vi "test TCX read (installed 71).vi"() -> ()   [LabVIEW 2011] (continued)
xmlns=\"http://www.garmin.com/xmlschemas/ActivityExtension/v2\"><Watts>102</Watts></TPX></Extensions></Trackpoint><Trackpoint><Time>2008-03-03T23:20:02Z</Time><Position><LatitudeDegrees>35.874903</LatitudeDegrees><LongitudeDegrees>-78.936135</LongitudeDegrees></Position><AltitudeMeters>84.253</AltitudeMeters><DistanceMeters>19044.637</DistanceMeters><Cadence>79</Cadence><Extensions><TPX xmlns=\"http://www.garmin.com/xmlschemas/ActivityExtension/v2\"><Watts>106</Watts></TPX></Extensions></Trackpoint><Trackpoint><Time>2008-03-03T23:20:03Z</Time><Position><LatitudeDegrees>35.874904</LatitudeDegrees><LongitudeDegrees>-78.936208</LongitudeDegrees></Position><AltitudeMeters>84.253</AltitudeMeters><DistanceMeters>19051.244</DistanceMeters><Cadence>79</Cadence><Extensions><TPX xmlns=\"http://www.garmin.com/xmlschemas/ActivityExtension/v2\"><Watts>107</Watts></TPX></Extensions></Trackpoint><Trackpoint><Time>2008-03-03T23:20:04Z</Time><Position><LatitudeDegrees>35.874906</LatitudeDegrees><LongitudeDegrees>-78.936282</LongitudeDegrees></Position><AltitudeMeters>84.253</AltitudeMeters><DistanceMeters>19057.943</DistanceMeters><Cadence>80</Cadence><Extensions><TPX xmlns=\"http://www.garmin.com/xmlschemas/ActivityExtension/v2\"><Watts>102</Watts></TPX></Extensions></Trackpoint><Trackpoint><Time>2008-03-03T23:20:05Z</Time><Position><LatitudeDegrees>35.874910</LatitudeDegrees><LongitudeDegrees>-78.936356</LongitudeDegrees></Position><AltitudeMeters>84.253</AltitudeMeters><DistanceMeters>19064.650</DistanceMeters><Cadence>80</Cadence><Extensions><TPX xmlns=\"http://www.garmin.com/xmlschemas/ActivityExtension/v2\"><Watts>102</Watts></TPX></Extensions></Trackpoint><Trackpoint><Time>2008-03-03T23:20:06Z</Time><Position><LatitudeDegrees>35.874914</LatitudeDegrees><LongitudeDegrees>-78.936430</LongitudeDegrees></Position><AltitudeMeters>84.253</AltitudeMeters><DistanceMeters>19071.314</DistanceMeters><Cadence>79</Cadence><Extensions><TPX xmlns=\"http://www.garmin.com/xmlschemas/ActivityExtension/v2\"><Watts>92</Watts></TPX></Extensions></Trackpoint><Trackpoint><Time>2008-03-03T23:20:07Z</Time><Position><LatitudeDegrees>35.874920</LatitudeDegrees><LongitudeDegrees>-78.936503</LongitudeDegrees></Position><AltitudeMeters>83.772</AltitudeMeters><DistanceMeters>19077.914</DistanceMeters><Cadence>81</Cadence><Extensions><TPX xmlns=\"http://www.garmin.com/xmlschemas/ActivityExtension/v2\"><Watts>82</Watts></TPX></Extensions></Trackpoint><Trackpoint><Time>2008-03-03T23:20:08Z</Time><Position><LatitudeDegrees>35.874928</LatitudeDegrees><LongitudeDegrees>-78.936576</LongitudeDegrees></Position><AltitudeMeters>84.253</AltitudeMeters><DistanceMeters>19084.633</DistanceMeters><Cadence>81</Cadence><Extensions><TPX xmlns=\"http://www.garmin.com/xmlschemas/ActivityExtension/v2\"><Watts>82</Watts></TPX></Extensions></Trackpoint><Trackpoint><Time>2008-03-03T23:20:09Z</Time><Position><LatitudeDegrees>35.874938</LatitudeDegrees><LongitudeDegrees>-78.936651</LongitudeDegrees></Position><AltitudeMeters>84.253</AltitudeMeters><DistanceMeters>19091.451</DistanceMeters><Cadence>83</Cadence><Extensions><TPX xmlns=\"http://www.garmin.com/xmlschemas/ActivityExtension/v2\"><Watts>76</Watts></TPX></Extensions></Trackpoint><Trackpoint><Time>2008-03-03T23:20:10Z</Time><Position><LatitudeDegrees>35.874950</LatitudeDegrees><LongitudeDegrees>-78.936725</LongitudeDegrees></Position><AltitudeMeters>83.772</AltitudeMeters><DistanceMeters>19098.295</DistanceMeters><Cadence>83</Cadence><Extensions><TPX xmlns=\"http://www.garmin.com/xmlschemas/ActivityExtension/v2\"><Watts>75</Watts></TPX></Extensions></Trackpoint><Trackpoint><Time>2008-03-03T23:20:11Z</Time><Position><LatitudeDegrees>35.874964</LatitudeDegrees><LongitudeDegrees>-78.936800</LongitudeDegrees></Position><AltitudeMeters>83.291</AltitudeMeters><DistanceMeters>19105.271</DistanceMeters><Cadence>84</Cadence><Extensions><TPX xmlns=\"http://www.garmin.com/xmlschemas/ActivityExtension/v2\"><Watts>68</Watts></TPX></Extensions></Trackpoint><Trackpoint><Time>2008-03-03T23:20:12Z</Time><Position><LatitudeDegrees>35.874981</LatitudeDegrees><LongitudeDegrees>-78.936875</LongitudeDegrees></Position><AltitudeMeters>83.772</AltitudeMeters><DistanceMeters>19112.254</DistanceMeters><Cadence>73</Cadence><Extensions><TPX xmlns=\"http://www.garmin.com/xmlschemas/ActivityExtension/v2\"><Watts>62</Watts></TPX></Extensions></Trackpoint><Trackpoint><Time>2008-03-03T23:20:13Z</Time><Position><LatitudeDegrees>35.875001</LatitudeDegrees><LongitudeDegrees>-78.936950</LongitudeDegrees></Position><AltitudeMeters>83.772</AltitudeMeters><DistanceMeters>19119.385</DistanceMeters><Cadence>73</Cadence><Extensions><TPX xmlns=\"http://www.garmin.com/xmlschemas/ActivityExtension/v2\"><Watts>61</Watts></TPX></Extensions></Trackpoint><Trackpoint><Time>2008-03-03T23:20:14Z</Time><Position><LatitudeDegrees>35.875020</LatitudeDegrees><LongitudeDegrees>-78.937025</LongitudeDegrees></Position><AltitudeMeters>83.772</AltitudeMeters><DistanceMeters>19126.529</DistanceMeters><Cadence>75</Cadence><Extensions><TPX xmlns=\"http://www.garmin.com/xmlschemas/ActivityExtension/v2\"><Watts>82</Watts></TPX></Extensions></Trackpoint><Trackpoint><Time>2008-03-03T23:20:15Z</Time><Position><LatitudeDegrees>35.875042</LatitudeDegrees><LongitudeDegrees>-78.937101</LongitudeDegrees></Position><AltitudeMeters>83.772</AltitudeMeters><DistanceMeters>19133.760</DistanceMeters><Cadence>77</Cadence><Extensions><TPX xmlns=\"http://www.garmin.com/xmlschemas/ActivityExtension/v2\"><Watts>83</Watts></TPX></Extensions></Trackpoint><Trackpoint><Time>2008-03-03T23:20:16Z</Time><Position><LatitudeDegrees>35.875070</LatitudeDegrees><LongitudeDegrees>-78.937176</LongitudeDegrees></Position><AltitudeMeters>83.291</AltitudeMeters><DistanceMeters>19141.281</DistanceMeters><Cadence>79</Cadence><Extensions><TPX xmlns=\"http://www.garmin.com/xmlschemas/ActivityExtension/v2\"><Watts>80</Watts></TPX></Extensions></Trackpoint><Trackpoint><Time>2008-03-03T23:20:17Z</Time><Position><LatitudeDegrees>35.875100</LatitudeDegrees><LongitudeDegrees>-78.937253</LongitudeDegrees></Position><AltitudeMeters>83.772</AltitudeMeters><DistanceMeters>19148.980</DistanceMeters><Cadence>80</Cadence><Extensions><TPX xmlns=\"http://www.garmin.com/xmlschemas/ActivityExtension/v2\"><Watts>77</Watts></TPX></Extensions></Trackpoint><Trackpoint><Time>2008-03-03T23:20:18Z</Time><Position><LatitudeDegrees>35.875133</LatitudeDegrees><LongitudeDegrees>-78.937330</LongitudeDegrees></Position><AltitudeMeters>83.291</AltitudeMeters><DistanceMeters>19156.816</DistanceMeters><Cadence>80</Cadence><Extensions><TPX xmlns=\"http://www.garmin.com/xmlschemas/ActivityExtension/v2\"><Watts>78</Watts></TPX></Extensions></Trackpoint><Trackpoint><Time>2008-03-03T23:20:19Z</Time><Position><LatitudeDegrees>35.875170</LatitudeDegrees><LongitudeDegrees>-78.937407</LongitudeDegrees></Position><AltitudeMeters>82.811</AltitudeMeters><DistanceMeters>19164.941</DistanceMeters><Cadence>83</Cadence><Extensions><TPX xmlns=\"http://www.garmin.com/xmlschemas/ActivityExtension/v2\"><Watts>56</Watts></TPX></Extensions></Trackpoint><Trackpoint><Time>2008-03-03T23:20:20Z</Time><Position><LatitudeDegrees>35.875210</LatitudeDegrees><LongitudeDegrees>-78.937487</LongitudeDegrees></Position><AltitudeMeters>82.811</AltitudeMeters><DistanceMeters>19173.371</DistanceMeters><Cadence>83</Cadence><Extensions><TPX xmlns=\"http://www.garmin.com/xmlschemas/ActivityExtension/v2\"><Watts>56</Watts></TPX></Extensions></Trackpoint><Trackpoint><Time>2008-03-03T23:20:21Z</Time><Position><LatitudeDegrees>35.875251</LatitudeDegrees><LongitudeDegrees>-78.937568</LongitudeDegrees></Position><AltitudeMeters>81.849</AltitudeMeters><DistanceMeters>19182.129</DistanceMeters><Cadence>74</Cadence><Extensions><TPX xmlns=\"http://www.garmin.com/xmlschemas/ActivityExtension/v2\"><Watts>48</Watts></TPX></Extensions></Trackpoint><Trackpoint><Time>2008-03-03T23:20:22Z</Time><Position><LatitudeDegrees>35.875295</LatitudeDegrees><LongitudeDegrees>-78.937653</LongitudeDegrees></Position><AltitudeMeters>81.369</AltitudeMeters><DistanceMeters>19191.217</DistanceMeters><Cadence>74</Cadence><Extensions><TPX xmlns=\"http://www.garmin.com/xmlschemas/ActivityExtension/v2\"><Watts>44</Watts></TPX></Extensions></Trackpoint><Trackpoint><Time>2008-03-03T23:20:23Z</Time><Position><LatitudeDegrees>35.875343</LatitudeDegrees><LongitudeDegrees>-78.937743</LongitudeDegrees></Position><AltitudeMeters>80.888</AltitudeMeters><DistanceMeters>19200.906</DistanceMeters><Cadence>79</Cadence><Extensions><TPX xmlns=\"http://www.garmin.com/xmlschemas/ActivityExtension/v2\"><Watts>47</Watts></TPX></Extensions></Trackpoint><Trackpoint><Time>2008-03-03T23:20:24Z</Time><Position><LatitudeDegrees>35.875392</LatitudeDegrees><LongitudeDegrees>-78.937838</LongitudeDegrees></Position><AltitudeMeters>80.888</AltitudeMeters><DistanceMeters>19211.127</DistanceMeters><Cadence>83</Cadence><Extensions><TPX xmlns=\"http://www.garmin.com/xmlschemas/ActivityExtension/v2\"><Watts>50</Watts></TPX></Extensions></Trackpoint><Trackpoint><Time>2008-03-03T23:20:25Z</Time><Position><LatitudeDegrees>35.875444</LatitudeDegrees><LongitudeDegrees>-78.937936</LongitudeDegrees></Position><AltitudeMeters>79.927</AltitudeMeters><DistanceMeters>19221.766</DistanceMeters><Cadence>87</Cadence><Extensions><TPX xmlns=\"http://www.garmin.com/xmlschemas/ActivityExtension/v2\"><Watts>50</Watts></TPX></Extensions></Trackpoint><Trackpoint><Time>2008-03-03T23:20:26Z</Time><Position><LatitudeDegrees>35.875500</LatitudeDegrees><LongitudeDegrees>-78.938041</LongitudeDegrees></Position><AltitudeMeters>78.965</AltitudeMeters><DistanceMeters>19233.037</DistanceMeters><Cadence>91</Cadence><Extensions><TPX xmlns=\"http://www.garmin.com/xmlschemas/ActivityExtension/v2\"><Watts>50</Watts></TPX></Extensions></Trackpoint><Trackpoint><Time>2008-03-03T23:20:27Z</Time><Position><LatitudeDegrees>35.875560</LatitudeDegrees><LongitudeDegrees>-78.938150</LongitudeDegrees></Position><AltitudeMeters>77.523</AltitudeMeters><DistanceMeters>19244.977</DistanceMeters><Cadence>91</Cadence><Extensions><TPX xmlns=\"http://www.garmin.com/xmlschemas/ActivityExtension/v2\"><Watts>48</Watts></TPX></Extensions></Trackpoint><Trackpoint><Time>2008-03-03T23:20:28Z</Time><Position><LatitudeDegrees>35.875621</LatitudeDegrees><LongitudeDegrees>-78.938266</LongitudeDegrees></Position><AltitudeMeters>77.523</AltitudeMeters><DistanceMeters>19257.467</DistanceMeters><Cadence>91</Cadence><Extensions><TPX xmlns=\"http://www.garmin.com/xmlschemas/ActivityExtension/v2\"><Watts>47</Watts></TPX></Extensions></Trackpoint><Trackpoint><Time>2008-03-03T23:20:29Z</Time><Position><LatitudeDegrees>35.875684</LatitudeDegrees><LongitudeDegrees>-78.938386</LongitudeDegrees></Position><AltitudeMeters>77.043</AltitudeMeters><DistanceMeters>19270.387</DistanceMeters><Cadence>93</Cadence><Extensions><TPX xmlns=\"http://www.garmin.com/xmlschemas/ActivityExtension/v2\"><Watts>54</Watts></TPX></Extensions></Trackpoint><Trackpoint><Time>2008-03-03T23:20:30Z</Time><Position><LatitudeDegrees>35.875749</LatitudeDegrees><LongitudeDegrees>-78.938510</LongitudeDegrees></Position><AltitudeMeters>76.081</AltitudeMeters><DistanceMeters>19283.744</DistanceMeters><Cadence>94</Cadence><Extensions><TPX xmlns=\"http://www.garmin.com/xmlschemas/ActivityExtension/v2\"><Watts>55</Watts></TPX></Extensions></Trackpoint><Trackpoint><Time>2008-03-03T23:20:31Z</Time><Position><LatitudeDegrees>35.875816</LatitudeDegrees><LongitudeDegrees>-78.938639</LongitudeDegrees></Position><AltitudeMeters>75.601</AltitudeMeters><DistanceMeters>19297.533</DistanceMeters><Cadence>98</Cadence><Extensions><TPX xmlns=\"http://www.garmin.com/xmlschemas/ActivityExtension/v2\"><Watts>62</Watts></TPX></Extensions></Trackpoint><Trackpoint><Time>2008-03-03T23:20:32Z</Time><Position><LatitudeDegrees>35.875883</LatitudeDegrees><LongitudeDegrees>-78.938771</LongitudeDegrees></Position><AltitudeMeters>73.198</AltitudeMeters><DistanceMeters>19311.721</DistanceMeters><Cadence>99</Cadence><Extensions><TPX xmlns=\"http://www.garmin.com/xmlschemas/ActivityExtension/v2\"><Watts>66</Watts></TPX></Extensions></Trackpoint><Trackpoint><Time>2008-03-03T23:20:33Z</Time><Position><LatitudeDegrees>35.875951</LatitudeDegrees><LongitudeDegrees>-78.938906</LongitudeDegrees></Position><AltitudeMeters>72.717</AltitudeMeters><DistanceMeters>19326.047</DistanceMeters><Cadence>100</Cadence><Extensions><TPX xmlns=\"http://www.garmin.com/xmlschemas/ActivityExtension/v2\"><Watts>74</Watts></TPX></Extensions></Trackpoint><Trackpoint><Time>2008-03-03T23:20:34Z</Time><Position><LatitudeDegrees>35.876019</LatitudeDegrees><LongitudeDegrees>-78.939044</LongitudeDegrees></Position><AltitudeMeters>72.717</AltitudeMeters><DistanceMeters>19340.588</DistanceMeters><Cadence>102</Cadence><Extensions><TPX xmlns=\"http://www.garmin.com/xmlschemas/ActivityExtension/v2\"><Watts>94</Watts></TPX></Extensions></Trackpoint><Trackpoint><Time>2008-03-03T23:20:35Z</Time><Position><LatitudeDegrees>35.876085</LatitudeDegrees><LongitudeDegrees>-78.939182</LongitudeDegrees></Position><AltitudeMeters>70.794</AltitudeMeters><DistanceMeters>19355.066</DistanceMeters><Cadence>102</Cadence><Extensions><TPX xmlns=\"http://www.garmin.com/xmlschemas/ActivityExtension/v2\"><Watts>94</Watts></TPX></Extensions></Trackpoint><Trackpoint><Time>2008-03-03T23:20:36Z</Time><Position><LatitudeDegrees>35.876149</LatitudeDegrees><LongitudeDegrees>-78.939320</LongitudeDegrees></Position><AltitudeMeters>71.275</AltitudeMeters><DistanceMeters>19369.359</DistanceMeters><Cadence>100</Cadence><Extensions><TPX xmlns=\"http://www.garmin.com/xmlschemas/ActivityExtension/v2\"><Watts>98</Watts></TPX></Extensions></Trackpoint><Trackpoint><Time>2008-03-03T23:20:37Z</Time><Position><LatitudeDegrees>35.876207</LatitudeDegrees><LongitudeDegrees>-78.939460</LongitudeDegrees></Position><AltitudeMeters>70.794</AltitudeMeters><DistanceMeters>19383.562</DistanceMeters><Cadence>99</Cadence><Extensions><TPX xmlns=\"http://www.garmin.com/xmlschemas/ActivityExtension/v2\"><Watts>92</Watts></TPX></Extensions></Trackpoint><Trackpoint><Time>2008-03-03T23:20:38Z</Time><Position><LatitudeDegrees>35.876256</LatitudeDegrees><LongitudeDegrees>-78.939603</LongitudeDegrees></Position><AltitudeMeters>69.352</AltitudeMeters><DistanceMeters>19397.516</DistanceMeters><Cadence>98</Cadence><Extensions><TPX xmlns=\"http://www.garmin.com/xmlschemas/ActivityExtension/v2\"><Watts>102</Watts></TPX></Extensions></Trackpoint><Trackpoint><Time>2008-03-03T23:20:39Z</Time><Position><LatitudeDegrees>35.876298</LatitudeDegrees><LongitudeDegrees>-78.939748</LongitudeDegrees></Position><AltitudeMeters>68.872</AltitudeMeters><DistanceMeters>19411.439</DistanceMeters><Cadence>98</Cadence><Extensions><TPX xmlns=\"http://www.garmin.com/xmlschemas/ActivityExtension/v2\"><Watts>99</Watts></TPX></Extensions></Trackpoint><Trackpoint><Time>2008-03-03T23:20:40Z</Time><Position><LatitudeDegrees>35.876331</LatitudeDegrees><LongitudeDegrees>-78.939897</LongitudeDegrees></Position><AltitudeMeters>68.391</AltitudeMeters><DistanceMeters>19425.348</DistanceMeters><Cadence>98</Cadence><Extensions><TPX xmlns=\"http://www.garmin.com/xmlschemas/ActivityExtension/v2\"><Watts>87</Watts></TPX></Extensions></Trackpoint><Trackpoint><Time>2008-03-03T23:20:41Z</Time><Position><LatitudeDegrees>35.876356</LatitudeDegrees><LongitudeDegrees>-78.940046</LongitudeDegrees></Position><AltitudeMeters>68.872</AltitudeMeters><DistanceMeters>19439.086</DistanceMeters><Cadence>97</Cadence><Extensions><TPX xmlns=\"http://www.garmin.com/xmlschemas/ActivityExtension/v2\"><Watts>87</Watts></TPX></Extensions></Trackpoint><Trackpoint><Time>2008-03-03T23:20:42Z</Time><Position><LatitudeDegrees>35.876377</LatitudeDegrees><LongitudeDegrees>-78.940195</LongitudeDegrees></Position><AltitudeMeters>67.910</AltitudeMeters><DistanceMeters>19452.791</DistanceMeters><Cadence>96</Cadence><Extensions><TPX xmlns=\"http://www.garmin.com/xmlschemas/ActivityExtension/v2\"><Watts>89</Watts></TPX></Extensions></Trackpoint><Trackpoint><Time>2008-03-03T23:20:43Z</Time><Position><LatitudeDegrees>35.876391</LatitudeDegrees><LongitudeDegrees>-78.940344</LongitudeDegrees></Position><AltitudeMeters>67.430</AltitudeMeters><DistanceMeters>19466.293</DistanceMeters><Cadence>94</Cadence><Extensions><TPX xmlns=\"http://www.garmin.com/xmlschemas/ActivityExtension/v2\"><Watts>100</Watts></TPX></Extensions></Trackpoint><Trackpoint><Time>2008-03-03T23:20:44Z</Time><Position><LatitudeDegrees>35.876400</LatitudeDegrees><LongitudeDegrees>-78.940524</LongitudeDegrees></Position><AltitudeMeters>67.430</AltitudeMeters><DistanceMeters>19482.514</DistanceMeters><Cadence>92</Cadence><Extensions><TPX xmlns=\"http://www.garmin.com/xmlschemas/ActivityExtension/v2\"><Watts>104</Watts></TPX></Extensions></Trackpoint><Trackpoint><Time>2008-03-03T23:20:45Z</Time><Position><LatitudeDegrees>35.876396</LatitudeDegrees><LongitudeDegrees>-78.940664</LongitudeDegrees></Position><AltitudeMeters>66.468</AltitudeMeters><DistanceMeters>19495.260</DistanceMeters><Cadence>90</Cadence><Extensions><TPX xmlns=\"http://www.garmin.com/xmlschemas/ActivityExtension/v2\"><Watts>104</Watts></TPX></Extensions></Trackpoint><Trackpoint><Time>2008-03-03T23:20:46Z</Time><Position><LatitudeDegrees>35.876381</LatitudeDegrees><LongitudeDegrees>-78.940801</LongitudeDegrees></Position><AltitudeMeters>66.949</AltitudeMeters><DistanceMeters>19507.684</DistanceMeters><Cadence>87</Cadence><Extensions><TPX xmlns=\"http://www.garmin.com/xmlschemas/ActivityExtension/v2\"><Watts>101</Watts></TPX></Extensions></Trackpoint><Trackpoint><Time>2008-03-03T23:20:47Z</Time><Position><LatitudeDegrees>35.876365</LatitudeDegrees><LongitudeDegrees>-78.940936</LongitudeDegrees></Position><AltitudeMeters>66.468</AltitudeMeters><DistanceMeters>19519.971</DistanceMeters><Cadence>86</Cadence><Extensions><TPX xmlns=\"http://www.garmin.com/xmlschemas/ActivityExtension/v2\"><Watts>97</Watts></TPX></Extensions></Trackpoint><Trackpoint><Time>2008-03-03T23:20:48Z</Time><Position><LatitudeDegrees>35.876347</LatitudeDegrees><LongitudeDegrees>-78.941069</LongitudeDegrees></Position><AltitudeMeters>66.468</AltitudeMeters><DistanceMeters>19532.281</DistanceMeters><Cadence>84</Cadence><Extensions><TPX xmlns=\"http://www.garmin.com/xmlschemas/ActivityExtension/v2\"><Watts>91</Watts></TPX></Extensions></Trackpoint><Trackpoint><Time>2008-03-03T23:20:49Z</Time><Position><LatitudeDegrees>35.876323</LatitudeDegrees><LongitudeDegrees>-78.941194</LongitudeDegrees></Position><AltitudeMeters>65.988</AltitudeMeters><DistanceMeters>19543.754</DistanceMeters><Cadence>83</Cadence><Extensions><TPX xmlns=\"http://www.garmin.com/xmlschemas/ActivityExtension/v2\"><Watts>98</Watts></TPX></Extensions></Trackpoint><Trackpoint><Time>2008-03-03T23:20:50Z</Time><Position><LatitudeDegrees>35.876300</LatitudeDegrees><LongitudeDegrees>-78.941319</LongitudeDegrees></Position><AltitudeMeters>65.988</AltitudeMeters><DistanceMeters>19555.248</DistanceMeters><Cadence>82</Cadence><Extensions><TPX xmlns=\"http://www.garmin.com/xmlschemas/ActivityExtension/v2\"><Watts>103</Watts></TPX></Extensions></Trackpoint><Trackpoint><Time>2008-03-03T23:20:51Z</Time><Position><LatitudeDegrees>35.876276</LatitudeDegrees><LongitudeDegrees>-78.941441</LongitudeDegrees></Position><AltitudeMeters>65.507</AltitudeMeters><DistanceMeters>19566.572</DistanceMeters><Cadence>81</Cadence><Extensions><TPX xmlns=\"http://www.garmin.com/xmlschemas/ActivityExtension/v2\"><Watts>102</Watts></TPX></Extensions></Trackpoint><Trackpoint><Time>2008-03-03T23:20:52Z</Time><Position><LatitudeDegrees>35.876255</LatitudeDegrees><LongitudeDegrees>-78.941561</LongitudeDegrees></Position><AltitudeMeters>65.507</AltitudeMeters><DistanceMeters>19577.674</DistanceMeters><Cadence>80</Cadence><Extensions><TPX xmlns=\"http://www.garmin.com/xmlschemas/ActivityExtension/v2\"><Watts>102</Watts></TPX></Extensions></Trackpoint><Trackpoint><Time>2008-03-03T23:20:53Z</Time><Position><LatitudeDegrees>35.876234</LatitudeDegrees><LongitudeDegrees>-78.941680</LongitudeDegrees></Position><AltitudeMeters>65.988</AltitudeMeters><DistanceMeters>19588.668</DistanceMeters><Cadence>79</Cadence><Extensions><TPX xmlns=\"http://www.garmin.com/xmlschemas/ActivityExtension/v2\"><Watts>104</Watts></TPX></Extensions></Trackpoint><Trackpoint><Time>2008-03-03T23:20:54Z</Time><Position><LatitudeDegrees>35.876210</LatitudeDegrees><LongitudeDegrees>-78.941800</LongitudeDegrees></Position><AltitudeMeters>65.507</AltitudeMeters><DistanceMeters>19599.725</DistanceMeters><Cadence>78</Cadence><Extensions><TPX xmlns=\"http://www.garmin.com/xmlschemas/ActivityExtension/v2\"><Watts>121</Watts></TPX></Extensions></Trackpoint><Trackpoint><Time>2008-03-03T23:20:55Z</Time><Position><LatitudeDegrees>35.876188</LatitudeDegrees><LongitudeDegrees>-78.941919</LongitudeDegrees></Position><AltitudeMeters>65.026</AltitudeMeters><DistanceMeters>19610.766</DistanceMeters><Cadence>79</Cadence><Extensions><TPX xmlns=\"http://www.garmin.com/xmlschemas/ActivityExtension/v2\"><Watts>128</Watts></TPX></Extensions></Trackpoint><Trackpoint><Time>2008-03-03T23:20:56Z</Time><Position><LatitudeDegrees>35.876169</LatitudeDegrees><LongitudeDegrees>-78.942040</LongitudeDegrees></Position><AltitudeMeters>65.026</AltitudeMeters><DistanceMeters>19622.070</DistanceMeters><Cadence>79</Cadence><Extensions><TPX xmlns=\"http://www.garmin.com/xmlschemas/ActivityExtension/v2\"><Watts>132</Watts></TPX></Extensions></Trackpoint><Trackpoint><Time>2008-03-03T23:20:57Z</Time><Position><LatitudeDegrees>35.876156</LatitudeDegrees><LongitudeDegrees>-78.942162</LongitudeDegrees></Position><AltitudeMeters>64.065</AltitudeMeters><DistanceMeters>19633.021</DistanceMeters><Cadence>79</Cadence><Extensions><TPX xmlns=\"http://www.garmin.com/xmlschemas/ActivityExtension/v2\"><Watts>129</Watts></TPX></Extensions></Trackpoint><Trackpoint><Time>2008-03-03T23:20:58Z</Time><Position><LatitudeDegrees>35.876143</LatitudeDegrees><LongitudeDegrees>-78.942283</LongitudeDegrees></Position><AltitudeMeters>64.065</AltitudeMeters><DistanceMeters>19644.061</DistanceMeters><Cadence>79</Cadence><Extensions><TPX xmlns=\"http://www.garmin.com/xmlschemas/ActivityExtension/v2\"><Watts>130</Watts></TPX></Extensions></Trackpoint><Trackpoint><Time>2008-03-03T23:20:59Z</Time><Position><LatitudeDegrees>35.876134</LatitudeDegrees><LongitudeDegrees>-78.942406</LongitudeDegrees></Position><AltitudeMeters>64.065</AltitudeMeters><DistanceMeters>19655.246</DistanceMeters><Cadence>79</Cadence><Extensions><TPX xmlns=\"http://www.garmin.com/xmlschemas/ActivityExtension/v2\"><Watts>131</Watts></TPX></Extensions></Trackpoint><Trackpoint><Time>2008-03-03T23:21:00Z</Time><Position><LatitudeDegrees>35.876123</LatitudeDegrees><LongitudeDegrees>-78.942528</LongitudeDegrees></Position><AltitudeMeters>64.065</AltitudeMeters><DistanceMeters>19666.287</DistanceMeters><Cadence>80</Cadence><Extensions><TPX xmlns=\"http://www.garmin.com/xmlschemas/ActivityExtension/v2\"><Watts>121</Watts></TPX></Extensions></Trackpoint><Trackpoint><Time>2008-03-03T23:21:01Z</Time><Position><LatitudeDegrees>35.876109</LatitudeDegrees><LongitudeDegrees>-78.942652</LongitudeDegrees></Position><AltitudeMeters>64.065</AltitudeMeters><DistanceMeters>19677.535</DistanceMeters><Cadence>80</Cadence><Extensions><TPX xmlns=\"http://www.garmin.com/xmlschemas/ActivityExtension/v2\"><Watts>111</Watts></TPX></Extensions></Trackpoint><Trackpoint><Time>2008-03-03T23:21:02Z</Time><Position><LatitudeDegrees>35.876101</LatitudeDegrees><LongitudeDegrees>-78.942771</LongitudeDegrees></Position><AltitudeMeters>63.584</AltitudeMeters><DistanceMeters>19688.404</DistanceMeters><Cadence>80</Cadence><Extensions><TPX xmlns=\"http://www.garmin.com/xmlschemas/ActivityExtension/v2\"><Watts>111</Watts></TPX></Extensions></Trackpoint><Trackpoint><Time>2008-03-03T23:21:03Z</Time><Position><LatitudeDegrees>35.876094</LatitudeDegrees><LongitudeDegrees>-78.942890</LongitudeDegrees></Position><AltitudeMeters>63.104</AltitudeMeters><DistanceMeters>19699.182</DistanceMeters><Cadence>79</Cadence><Extensions><TPX xmlns=\"http://www.garmin.com/xmlschemas/ActivityExtension/v2\"><Watts>112</Watts></TPX></Extensions></Trackpoint><Trackpoint><Time>2008-03-03T23:21:04Z</Time><Position><LatitudeDegrees>35.876086</LatitudeDegrees><LongitudeDegrees>-78.943011</LongitudeDegrees></Position><AltitudeMeters>63.104</AltitudeMeters><DistanceMeters>19710.023</DistanceMeters><Cadence>78</Cadence><Extensions><TPX xmlns=\"http://www.garmin.com/xmlschemas/ActivityExtension/v2\"><Watts>113</Watts></TPX></Extensions></Trackpoint><Trackpoint><Time>2008-03-03T23:21:05Z</Time><Position><LatitudeDegrees>35.876087</LatitudeDegrees><LongitudeDegrees>-78.943132</LongitudeDegrees></Position><AltitudeMeters>64.065</AltitudeMeters><DistanceMeters>19721.125</DistanceMeters><Cadence>77</Cadence><Extensions><TPX xmlns=\"http://www.garmin.com/xmlschemas/ActivityExtension/v2\"><Watts>115</Watts></TPX></Extensions></Trackpoint><Trackpoint><Time>2008-03-03T23:21:06Z</Time><Position><LatitudeDegrees>35.876092</LatitudeDegrees><LongitudeDegrees>-78.943252</LongitudeDegrees></Position><AltitudeMeters>64.546</AltitudeMeters><DistanceMeters>19731.799</DistanceMeters><Cadence>75</Cadence><Extensions><TPX xmlns=\"http://www.garmin.com/xmlschemas/ActivityExtension/v2\"><Watts>131</Watts></TPX></Extensions></Trackpoint><Trackpoint><Time>2008-03-03T23:21:07Z</Time><Position><LatitudeDegrees>35.876092</LatitudeDegrees><LongitudeDegrees>-78.943365</LongitudeDegrees></Position><AltitudeMeters>64.065</AltitudeMeters><DistanceMeters>19742.010</DistanceMeters><Cadence>75</Cadence><Extensions><TPX xmlns=\"http://www.garmin.com/xmlschemas/ActivityExtension/v2\"><Watts>129</Watts></TPX></Extensions></Trackpoint><Trackpoint><Time>2008-03-03T23:21:08Z</Time><Position><LatitudeDegrees>35.876092</LatitudeDegrees><LongitudeDegrees>-78.943476</LongitudeDegrees></Position><AltitudeMeters>63.584</AltitudeMeters><DistanceMeters>19752.037</DistanceMeters><Cadence>73</Cadence><Extensions><TPX xmlns=\"http://www.garmin.com/xmlschemas/ActivityExtension/v2\"><Watts>138</Watts></TPX></Extensions></Trackpoint><Trackpoint><Time>2008-03-03T23:21:09Z</Time><Position><LatitudeDegrees>35.876096</LatitudeDegrees><LongitudeDegrees>-78.943589</LongitudeDegrees></Position><AltitudeMeters>64.065</AltitudeMeters><DistanceMeters>19762.207</DistanceMeters><Cadence>72</Cadence><Extensions><TPX xmlns=\"http://www.garmin.com/xmlschemas/ActivityExtension/v2\"><Watts>137</Watts></TPX></Extensions></Trackpoint><Trackpoint><Time>2008-03-03T23:21:10Z</Time><Position><LatitudeDegrees>35.876098</LatitudeDegrees><LongitudeDegrees>-78.943697</LongitudeDegrees></Position><AltitudeMeters>64.065</AltitudeMeters><DistanceMeters>19771.961</DistanceMeters><Cadence>70</Cadence><Extensions><TPX xmlns=\"http://www.garmin.com/xmlschemas/ActivityExtension/v2\"><Watts>135</Watts></TPX></Extensions></Trackpoint><Trackpoint><Time>2008-03-03T23:21:11Z</Time><Position><LatitudeDegrees>35.876103</LatitudeDegrees><LongitudeDegrees>-78.943804</LongitudeDegrees></Position><AltitudeMeters>63.584</AltitudeMeters><DistanceMeters>19781.617</DistanceMeters><Cadence>68</Cadence><Extensions><TPX xmlns=\"http://www.garmin.com/xmlschemas/ActivityExtension/v2\"><Watts>132</Watts></TPX></Extensions></Trackpoint><Trackpoint><Time>2008-03-03T23:21:12Z</Time><Position><LatitudeDegrees>35.876106</LatitudeDegrees><LongitudeDegrees>-78.943908</LongitudeDegrees></Position><AltitudeMeters>64.065</AltitudeMeters><DistanceMeters>19791.057</DistanceMeters><Cadence>71</Cadence><Extensions><TPX xmlns=\"http://www.garmin.com/xmlschemas/ActivityExtension/v2\"><Watts>122</Watts></TPX></Extensions></Trackpoint><Trackpoint><Time>2008-03-03T23:21:13Z</Time><Position><LatitudeDegrees>35.876106</LatitudeDegrees><LongitudeDegrees>-78.944009</LongitudeDegrees></Position><AltitudeMeters>64.065</AltitudeMeters><DistanceMeters>19800.074</DistanceMeters><Cadence>71</Cadence><Extensions><TPX xmlns=\"http://www.garmin.com/xmlschemas/ActivityExtension/v2\"><Watts>91</Watts></TPX></Extensions></Trackpoint><Trackpoint><Time>2008-03-03T23:21:14Z</Time><Position><LatitudeDegrees>35.876105</LatitudeDegrees><LongitudeDegrees>-78.944107</LongitudeDegrees></Position><AltitudeMeters>64.065</AltitudeMeters><DistanceMeters>19808.879</DistanceMeters><Cadence>76</Cadence><Extensions><TPX xmlns=\"http://www.garmin.com/xmlschemas/ActivityExtension/v2\"><Watts>60</Watts></TPX></Extensions></Trackpoint><Trackpoint><Time>2008-03-03T23:21:15Z</Time><Position><LatitudeDegrees>35.876107</LatitudeDegrees><LongitudeDegrees>-78.944199</LongitudeDegrees></Position><AltitudeMeters>64.546</AltitudeMeters><DistanceMeters>19817.195</DistanceMeters><Cadence>79</Cadence><Extensions><TPX xmlns=\"http://www.garmin.com/xmlschemas/ActivityExtension/v2\"><Watts>61</Watts></TPX></Extensions></Trackpoint><Trackpoint><Time>2008-03-03T23:21:16Z</Time><Position><LatitudeDegrees>35.876111</LatitudeDegrees><LongitudeDegrees>-78.944289</LongitudeDegrees></Position><AltitudeMeters>64.546</AltitudeMeters><DistanceMeters>19825.371</DistanceMeters><Cadence>77</Cadence><Extensions><TPX xmlns=\"http://www.garmin.com/xmlschemas/ActivityExtension/v2\"><Watts>103</Watts></TPX></Extensions></Trackpoint><Trackpoint><Time>2008-03-03T23:21:17Z</Time><Position><LatitudeDegrees>35.876114</LatitudeDegrees><LongitudeDegrees>-78.944379</LongitudeDegrees></Position><AltitudeMeters>65.026</AltitudeMeters><DistanceMeters>19833.463</DistanceMeters><Cadence>75</Cadence><Extensions><TPX xmlns=\"http://www.garmin.com/xmlschemas/ActivityExtension/v2\"><Watts>153</Watts></TPX></Extensions></Trackpoint><Trackpoint><Time>2008-03-03T23:21:18Z</Time><Position><LatitudeDegrees>35.876114</LatitudeDegrees><LongitudeDegrees>-78.944469</LongitudeDegrees></Position><AltitudeMeters>65.507</AltitudeMeters><DistanceMeters>19841.531</DistanceMeters><Cadence>74</Cadence><Extensions><TPX xmlns=\"http://www.garmin.com/xmlschemas/ActivityExtension/v2\"><Watts>219</Watts></TPX></Extensions></Trackpoint><Trackpoint><Time>2008-03-03T23:21:19Z</Time><Position><LatitudeDegrees>35.876113</LatitudeDegrees><LongitudeDegrees>-78.944557</LongitudeDegrees></Position><AltitudeMeters>65.507</AltitudeMeters><DistanceMeters>19849.498</DistanceMeters><Cadence>74</Cadence><Extensions><TPX xmlns=\"http://www.garmin.com/xmlschemas/ActivityExtension/v2\"><Watts>218</Watts></TPX></Extensions></Trackpoint><Trackpoint><Time>2008-03-03T23:21:20Z</Time><Position><LatitudeDegrees>35.876117</LatitudeDegrees><LongitudeDegrees>-78.944644</LongitudeDegrees></Position><AltitudeMeters>65.507</AltitudeMeters><DistanceMeters>19857.428</DistanceMeters><Cadence>73</Cadence><Extensions><TPX xmlns=\"http://www.garmin.com/xmlschemas/ActivityExtension/v2\"><Watts>288</Watts></TPX></Extensions></Trackpoint><Trackpoint><Time>2008-03-03T23:21:21Z</Time><Position><LatitudeDegrees>35.876123</LatitudeDegrees><LongitudeDegrees>-78.944730</LongitudeDegrees></Position><AltitudeMeters>65.988</AltitudeMeters><DistanceMeters>19865.123</DistanceMeters><Cadence>72</Cadence><Extensions><TPX xmlns=\"http://www.garmin.com/xmlschemas/ActivityExtension/v2\"><Watts>304</Watts></TPX></Extensions></Trackpoint><Trackpoint><Time>2008-03-03T23:21:22Z</Time><Position><LatitudeDegrees>35.876124</LatitudeDegrees><LongitudeDegrees>-78.944814</LongitudeDegrees></Position><AltitudeMeters>65.988</AltitudeMeters><DistanceMeters>19872.686</DistanceMeters><Cadence>72</Cadence><Extensions><TPX xmlns=\"http://www.garmin.com/xmlschemas/ActivityExtension/v2\"><Watts>285</Watts></TPX></Extensions></Trackpoint><Trackpoint><Time>2008-03-03T23:21:23Z</Time><Position><LatitudeDegrees>35.876125</LatitudeDegrees><LongitudeDegrees>-78.944898</LongitudeDegrees></Position><AltitudeMeters>65.988</AltitudeMeters><DistanceMeters>19880.324</DistanceMeters><Cadence>70</Cadence><Extensions><TPX xmlns=\"http://www.garmin.com/xmlschemas/ActivityExtension/v2\"><Watts>291</Watts></TPX></Extensions></Trackpoint><Trackpoint><Time>2008-03-03T23:21:24Z</Time><Position><LatitudeDegrees>35.876129</LatitudeDegrees><LongitudeDegrees>-78.944982</LongitudeDegrees></Position><AltitudeMeters>66.468</AltitudeMeters><DistanceMeters>19887.838</DistanceMeters><Cadence>70</Cadence><Extensions><TPX xmlns=\"http://www.garmin.com/xmlschemas/ActivityExtension/v2\"><Watts>291</Watts></TPX></Extensions></Trackpoint><Trackpoint><Time>2008-03-03T23:21:25Z</Time><Position><LatitudeDegrees>35.876133</LatitudeDegrees><LongitudeDegrees>-78.945064</LongitudeDegrees></Position><AltitudeMeters>66.949</AltitudeMeters><DistanceMeters>19895.252</DistanceMeters><Cadence>68</Cadence><Extensions><TPX xmlns=\"http://www.garmin.com/xmlschemas/ActivityExtension/v2\"><Watts>301</Watts></TPX></Extensions></Trackpoint><Trackpoint><Time>2008-03-03T23:21:26Z</Time><Position><LatitudeDegrees>35.876134</LatitudeDegrees><LongitudeDegrees>-78.945144</LongitudeDegrees></Position><AltitudeMeters>66.949</AltitudeMeters><DistanceMeters>19902.514</DistanceMeters><Cadence>68</Cadence><Extensions><TPX xmlns=\"http://www.garmin.com/xmlschemas/ActivityExtension/v2\"><Watts>324</Watts></TPX></Extensions></Trackpoint><Trackpoint><Time>2008-03-03T23:21:27Z</Time><Position><LatitudeDegrees>35.876136</LatitudeDegrees><LongitudeDegrees>-78.945225</LongitudeDegrees></Position><AltitudeMeters>67.430</AltitudeMeters><DistanceMeters>19909.877</DistanceMeters><Cadence>68</Cadence><Extensions><TPX xmlns=\"http://www.garmin.com/xmlschemas/ActivityExtension/v2\"><Watts>334</Watts></TPX></Extensions></Trackpoint><Trackpoint><Time>2008-03-03T23:21:28Z</Time><Position><LatitudeDegrees>35.876141</LatitudeDegrees><LongitudeDegrees>-78.945306</LongitudeDegrees></Position><AltitudeMeters>67.910</AltitudeMeters><DistanceMeters>19917.148</DistanceMeters><Cadence>68</Cadence><Extensions><TPX xmlns=\"http://www.garmin.com/xmlschemas/ActivityExtension/v2\"><Watts>357</Watts></TPX></Extensions></Trackpoint><Trackpoint><Time>2008-03-03T23:21:29Z</Time><Position><LatitudeDegrees>35.876147</LatitudeDegrees><LongitudeDegrees>-78.945389</LongitudeDegrees></Position><AltitudeMeters>67.910</AltitudeMeters><DistanceMeters>19924.643</DistanceMeters><Cadence>69</Cadence><Extensions><TPX xmlns=\"http://www.garmin.com/xmlschemas/ActivityExtension/v2\"><Watts>379</Watts></TPX></Extensions></Trackpoint><Trackpoint><Time>2008-03-03T23:21:30Z</Time><Position><LatitudeDegrees>35.876152</LatitudeDegrees><LongitudeDegrees>-78.945472</LongitudeDegrees></Position><AltitudeMeters>67.910</AltitudeMeters><DistanceMeters>19932.154</DistanceMeters><Cadence>71</Cadence><Extensions><TPX xmlns=\"http://www.garmin.com/xmlschemas/ActivityExtension/v2\"><Watts>448</Watts></TPX></Extensions></Trackpoint><Trackpoint><Time>2008-03-03T23:21:31Z</Time><Position><LatitudeDegrees>35.876154</LatitudeDegrees><LongitudeDegrees>-78.945555</LongitudeDegrees></Position><AltitudeMeters>68.391</AltitudeMeters><DistanceMeters>19939.660</DistanceMeters><Cadence>73</Cadence><Extensions><TPX xmlns=\"http://www.garmin.com/xmlschemas/ActivityExtension/v2\"><Watts>467</Watts></TPX></Extensions></Trackpoint><Trackpoint><Time>2008-03-03T23:21:32Z</Time><Position><LatitudeDegrees>35.876157</LatitudeDegrees><LongitudeDegrees>-78.945641</LongitudeDegrees></Position><AltitudeMeters>68.872</AltitudeMeters><DistanceMeters>19947.496</DistanceMeters><Cadence>73</Cadence><Extensions><TPX xmlns=\"http://www.garmin.com/xmlschemas/ActivityExtension/v2\"><Watts>465</Watts></TPX></Extensions></Trackpoint><Trackpoint><Time>2008-03-03T23:21:33Z</Time><Position><LatitudeDegrees>35.876158</LatitudeDegrees><LongitudeDegrees>-78.945725</LongitudeDegrees></Position><AltitudeMeters>68.872</AltitudeMeters><DistanceMeters>19955.113</DistanceMeters><Cadence>73</Cadence><Extensions><TPX xmlns=\"http://www.garmin.com/xmlschemas/ActivityExtension/v2\"><Watts>441</Watts></TPX></Extensions></Trackpoint><Trackpoint><Time>2008-03-03T23:21:34Z</Time><Position><LatitudeDegrees>35.876159</LatitudeDegrees><LongitudeDegrees>-78.945809</LongitudeDegrees></Position><AltitudeMeters>68.872</AltitudeMeters><DistanceMeters>19962.701</DistanceMeters><Cadence>74</Cadence><Extensions><TPX xmlns=\"http://www.garmin.com/xmlschemas/ActivityExtension/v2\"><Watts>443</Watts></TPX></Extensions></Trackpoint><Trackpoint><Time>2008-03-03T23:21:35Z</Time><Position><LatitudeDegrees>35.876160</LatitudeDegrees><LongitudeDegrees>-78.945896</LongitudeDegrees></Position><AltitudeMeters>68.872</AltitudeMeters><DistanceMeters>19970.531</DistanceMeters><Cadence>76</Cadence><Extensions><TPX xmlns=\"http://www.garmin.com/xmlschemas/ActivityExtension/v2\"><Watts>440</Watts></TPX></Extensions></Trackpoint><Trackpoint><Time>2008-03-03T23:21:36Z</Time><Position><LatitudeDegrees>35.876163</LatitudeDegrees><LongitudeDegrees>-78.945987</LongitudeDegrees></Position><AltitudeMeters>69.352</AltitudeMeters><DistanceMeters>19978.740</DistanceMeters><Cadence>76</Cadence><Extensions><TPX xmlns=\"http://www.garmin.com/xmlschemas/ActivityExtension/v2\"><Watts>437</Watts></TPX></Extensions></Trackpoint><Trackpoint><Time>2008-03-03T23:21:37Z</Time><Position><LatitudeDegrees>35.876167</LatitudeDegrees><LongitudeDegrees>-78.946079</LongitudeDegrees></Position><AltitudeMeters>69.352</AltitudeMeters><DistanceMeters>19987.109</DistanceMeters><Cadence>77</Cadence><Extensions><TPX xmlns=\"http://www.garmin.com/xmlschemas/ActivityExtension/v2\"><Watts>456</Watts></TPX></Extensions></Trackpoint><Trackpoint><Time>2008-03-03T23:21:38Z</Time><Position><LatitudeDegrees>35.876171</LatitudeDegrees><LongitudeDegrees>-78.946173</LongitudeDegrees></Position><AltitudeMeters>70.313</AltitudeMeters><DistanceMeters>19995.613</DistanceMeters><Cadence>81</Cadence><Extensions><TPX xmlns=\"http://www.garmin.com/xmlschemas/ActivityExtension/v2\"><Watts>438</Watts></TPX></Extensions></Trackpoint><Trackpoint><Time>2008-03-03T23:21:39Z</Time><Position><LatitudeDegrees>35.876177</LatitudeDegrees><LongitudeDegrees>-78.946269</LongitudeDegrees></Position><AltitudeMeters>70.313</AltitudeMeters><DistanceMeters>20004.225</DistanceMeters><Cadence>81</Cadence><Extensions><TPX xmlns=\"http://www.garmin.com/xmlschemas/ActivityExtension/v2\"><Watts>441</Watts></TPX></Extensions></Trackpoint><Trackpoint><Time>2008-03-03T23:21:40Z</Time><Position><LatitudeDegrees>35.876181</LatitudeDegrees><LongitudeDegrees>-78.946364</LongitudeDegrees></Position><AltitudeMeters>70.794</AltitudeMeters><DistanceMeters>20012.861</DistanceMeters><Cadence>77</Cadence><Extensions><TPX xmlns=\"http://www.garmin.com/xmlschemas/ActivityExtension/v2\"><Watts>382</Watts></TPX></Extensions></Trackpoint><Trackpoint><Time>2008-03-03T23:21:41Z</Time><Position><LatitudeDegrees>35.876188</LatitudeDegrees><LongitudeDegrees>-78.946455</LongitudeDegrees></Position><AltitudeMeters>71.275</AltitudeMeters><DistanceMeters>20021.104</DistanceMeters><Cadence>74</Cadence><Extensions><TPX xmlns=\"http://www.garmin.com/xmlschemas/ActivityExtension/v2\"><Watts>270</Watts></TPX></Extensions></Trackpoint><Trackpoint><Time>2008-03-03T23:21:42Z</Time><Position><LatitudeDegrees>35.876192</LatitudeDegrees><LongitudeDegrees>-78.946543</LongitudeDegrees></Position><AltitudeMeters>71.275</AltitudeMeters><DistanceMeters>20029.039</DistanceMeters><Cadence>72</Cadence><Extensions><TPX xmlns=\"http://www.garmin.com/xmlschemas/ActivityExtension/v2\"><Watts>185</Watts></TPX></Extensions></Trackpoint><Trackpoint><Time>2008-03-03T23:21:43Z</Time><Position><LatitudeDegrees>35.876191</LatitudeDegrees><LongitudeDegrees>-78.946626</LongitudeDegrees></Position><AltitudeMeters>71.275</AltitudeMeters><DistanceMeters>20036.525</DistanceMeters><Cadence>69</Cadence><Extensions><TPX xmlns=\"http://www.garmin.com/xmlschemas/ActivityExtension/v2\"><Watts>177</Watts></TPX></Extensions></Trackpoint><Trackpoint><Time>2008-03-03T23:21:44Z</Time><Position><LatitudeDegrees>35.876192</LatitudeDegrees><LongitudeDegrees>-78.946709</LongitudeDeg
